vi "Template.vi"(0 "PDF Report IN":refnum<class "PDF Report Class.lvclass">, 11 "error in (no error)":errorcluster) -> (4 "PDF Report OUT":refnum<class "PDF Report Class.lvclass">, 15 "error out":errorcluster)   [LabVIEW 2019]
doc: "Version 1.1\nDeveloped by Jean-Marc Simard\nCopyright © 2012, Exaprom Inc.\nAll rights reserved.\nLicense: BSD\n\nWith iTextSharp 4.1.6 (http://itextsharp.sourceforge.net)\nunder Mozilla Public License Version 1.1\n(http://www.mozilla.org/MPL/MPL-1.1.html)"
uses:
  <userlib>/Exaprom PDF/LV Class/PDF Report Class/PDF Report Class.lvclass
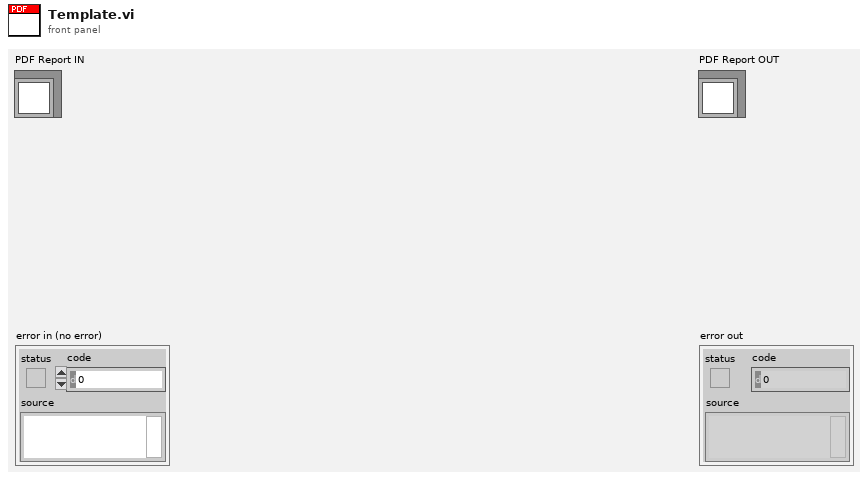
[diagram p1: front panel]
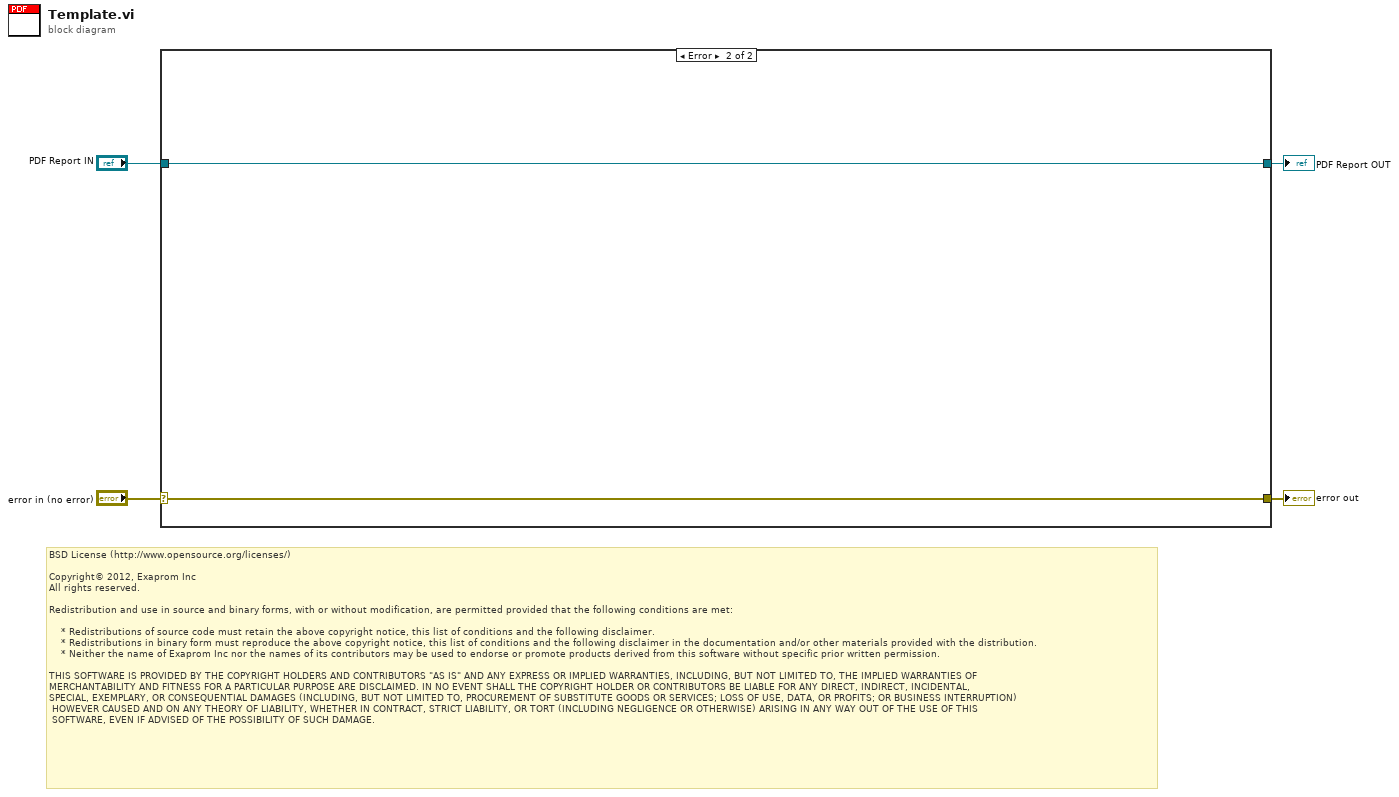
[diagram p0: block diagram]
diagram:
  # "BSD License (http://www.opensource.org/licenses/)\n\nCopyright© 2012, Exaprom Inc\nAll rights reserved.\n\nRedistribution and use in source and binary forms, with or without modification, are permitted provided that the following conditions are met:\n\n    * Redistributions of source code must retain the above copyright notice, this list of conditions and the following disclaimer.\n    * Redistributions in binary form must reproduce the above copyright notice, this list of conditions and the following disclaimer in the documentation and/or other materials provided with the distribution.\n    * Neither the name of Exaprom Inc nor the names of its contributors may be used to endorse or promote products derived from this software without specific prior written permission.\n\nTHIS SOFTWARE IS PROVIDED BY THE COPYRIGHT HOLDERS AND CONTRIBUTORS \"AS IS\" AND ANY EXPRESS OR IMPLIED WARRANTIES, INCLUDING, BUT NOT LIMITED TO, THE IMPLIED WARRANTIES OF \nMERCHANTABILITY AND FITNESS FOR A PARTICULAR PURPOSE ARE DISCLAIMED. IN NO EVENT SHALL THE COPYRIGHT HOLDER OR CONTRIBUTORS BE LIABLE FOR ANY DIRECT, INDIRECT, INCIDENTAL,\nSPECIAL, EXEMPLARY, OR CONSEQUENTIAL DAMAGES (INCLUDING, BUT NOT LIMITED TO, PROCUREMENT OF SUBSTITUTE GOODS OR SERVICES; LOSS OF USE, DATA, OR PROFITS; OR BUSINESS INTERRUPTION)\n HOWEVER CAUSED AND ON ANY THEORY OF LIABILITY, WHETHER IN CONTRACT, STRICT LIABILITY, OR TORT (INCLUDING NEGLIGENCE OR OTHERWISE) ARISING IN ANY WAY OUT OF THE USE OF THIS\n SOFTWARE, EVEN IF ADVISED OF THE POSSIBILITY OF SUCH DAMAGE."
  n1 = case shown="Error" "error in (no error)" {
    selector: "error in (no error)" -> [w5 w8]
    tunnel: "PDF Report IN" -> [w6 w7]
    tunnel: [w6 w7] -> w3
    tunnel: [w5 w8] -> w2
    frame No Error {
    }
    frame Error {
    }
  }
  "PDF Report OUT" <- w3
  "error out" <- w2
